vi "Create_Simple_DO_Signal.vi"(8 "error in":errorcluster, 9 "On/Off":bool, 10 "Samples / s (10000)":u32=10000, 11 "Time (s)":dbl=0.1) -> (0 "error out":errorcluster, 3 "Signal":u32[](array[numeric]))   [LabVIEW 2021]
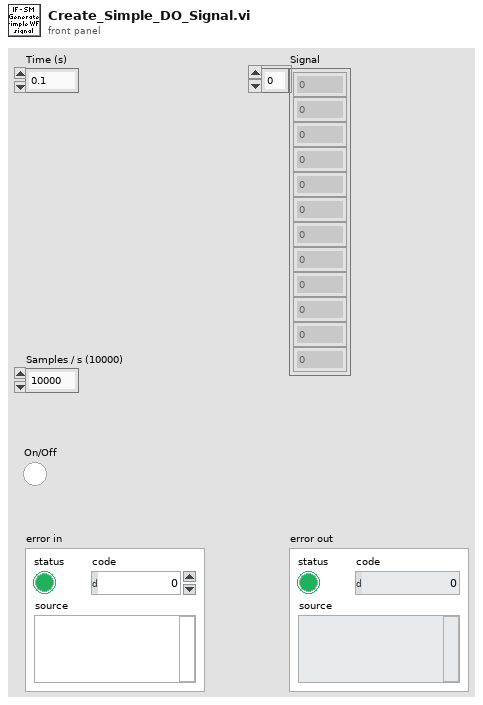
[diagram p1: front panel]
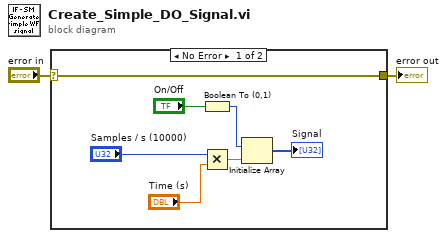
[diagram p0: block diagram]
diagram:
  n1 = case shown="No Error" "error in" {
    selector: "error in" -> [w4 w10]
    tunnel: [w4 w10] -> w1
    frame No Error {
      n2 = Boolean To (0,1)(Boolean="On/Off") -> (0, 1=w5:i16)
      n3 = Multiply(x="Samples / s (10000)", y="Time (s)") -> (x*y=w7:dbl)
      n4 = Initialize Array(w5, w7) -> (→"Signal":i16[])
    }
    frame Error {
    }
  }
  "error out" <- w1
